vi "serialization tests.vi"() -> ()   [LabVIEW 2013, in "Shared Library Module tests.lvlib"]
doc: "Platypus Framework 1.0.1.60\nNI Systems Engineering - National Instruments"
uses:
  Shared Library Module tests.lvlib
  <vilib>/NI/Tag Bus Module Framework/channel/channel classification.ctl
  configuration/Shared Library Module configuration.lvclass
  <vilib>/NI/Tag Bus Module Framework/channel/TBM channel.lvclass
  <vilib>/NI/Tag Bus Module Framework/root configuration/TBM configuration.lvclass
panel:
  out "channels equal":bool
  out "no error":errorcluster
  out "no error":errorcluster
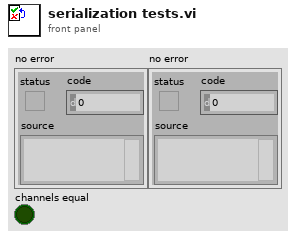
[diagram p1: front panel]
types:
  T1 = typedef "TBM channel.lvclass/channel classification.ctl" = enum16{"input data", "output data", "processing parameter", "processing result"}
  T2 = typedef "tag bus.lvlib/tag descriptor.lvclass/Data Type.ctl" = enum16{"Double", "Single", "I64", "I32", "I16", "I8", "U64", "U32", "U16", "U8", "Boolean", "String", "Array of Double", "Array of Single", "Array of I64", "Array of I32", "Array of I16", "Array of I8", "Array of U64", "Array of U32", "Array of U16", "Array of U8", "Array of Boolean", "Array of String"}
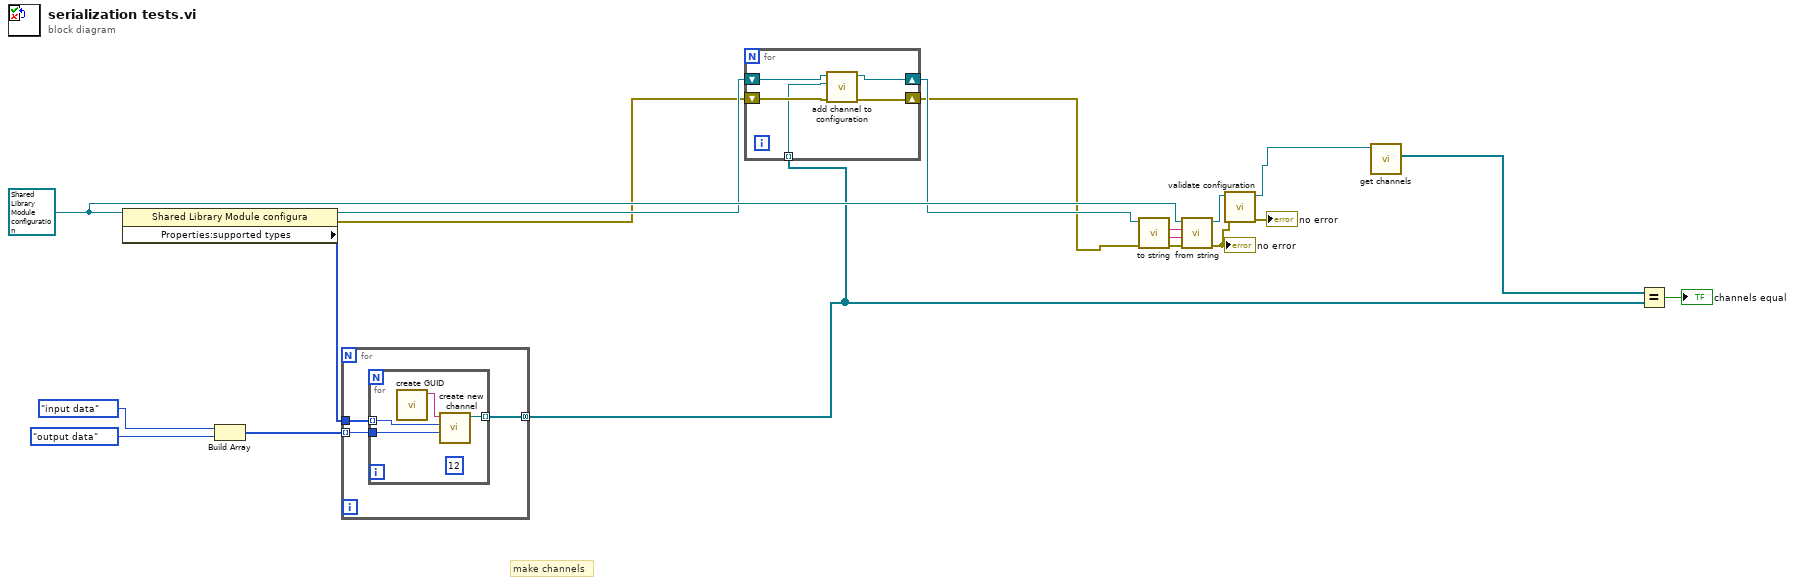
[diagram p0: block diagram]
diagram:
  w8 = refnum<class "Shared Library Module configuration.lvclass"> refnum ("tag bus configurable plugin module configuration")
  # "make channels"
  n1 = property class="Shared Library Module configura"(reference=w8) -> (reference out=w7:refnum<class "Shared Library Module configuration.lvclass">, error out=w4:errorcluster, "Properties:supported types"=w11:T2[])  [unwired: 1 in]
  n2 = Build Array(channel_classification."input data" ("channel classification"), channel_classification."output data" ("channel classification")) -> (w12:T1[])
  n3 = for {
    tunnel: w12 -> [w22] mode=indexing
    tunnel: [w21] -> w3 mode=concatenating
    tunnel: w11 -> [w20]
    n4 = for {
      tunnel: w22 -> [w25]
      tunnel: [w26] -> w21 mode=indexing
      tunnel: w20 -> [w24] mode=indexing
      (unwired) 12
      n5 = call <vilib>:"create GUID.vi"() -> ("uuid"=w23:string)  [unwired: 11 in]
      n6 = call <vilib>:"create new channel.vi"("channel classification"=w25, "data type"=w24, "channel name"=w23) -> ("channel"=w26:refnum<class "TBM channel.lvclass">)  [unwired: 8 in]
    }
  }
  n7 = for {
    shift-right: [w30] -> w6
    shift-left: w7 -> [w31]
    shift-right: [w29] -> w5
    shift-left: w4 -> [w28]
    tunnel: w3 -> [w27] mode=indexing
    n8 = call "add channel to configuration.vi"("error in"=w28, "TBM channel in"=w27, "Shared Library Module configuration in"=w31) -> ("error out"=w29:errorcluster, "Shared Library Module configuration out"=w30:refnum<class "Shared Library Module configuration.lvclass">)  [unwired: 7 in]
  }
  n9 = call-dynamic "to string.vi"("error in"=w5, "Shared Library Module configuration in"=w6) -> ("error out"=w19:errorcluster, "data"=w18:string, "version"=w17:string)  [unwired: 6 in, 1 out]
  n10 = call-dynamic "from string.vi"("error in"=w19, "data"=w18, "version"=w17, "Shared Library Module configuration in"=w8) -> ("error out"=w10:errorcluster, "Shared Library Module configuration out"=w16:refnum<class "Shared Library Module configuration.lvclass">)  [unwired: 6 in]
  "no error" <- w10
  n11 = call-dynamic "validate configuration.vi"("error in"=w10, "Shared Library Module configuration in"=w16) -> ("error out"=→"no error":errorcluster, "Shared Library Module configuration out"=w2:refnum<class "Shared Library Module configuration.lvclass">)  [unwired: 8 in]
  n12 = call-dynamic "get channels.vi"("Shared Library Module configuration in"=w2) -> ("channels"=w1:refnum<class "TBM channel.lvclass">[])  [unwired: 9 in, 1 out]
  n13 = Equal?(x=w1, y=w3) -> (x = y?=→"channels equal":bool)
